vi "encoding_matlab_guoy.vi"(0 "Encoding":cluster{"d":dbl, "y0":dbl, "y1":dbl}) -> (1 "l":dbl[](array[numeric]), 2 "p":dbl[](array[numeric]), 3 "coeffs":dbl[](array[numeric]), 4 "phase":dbl[](array[numeric]))   [LabVIEW 2015]
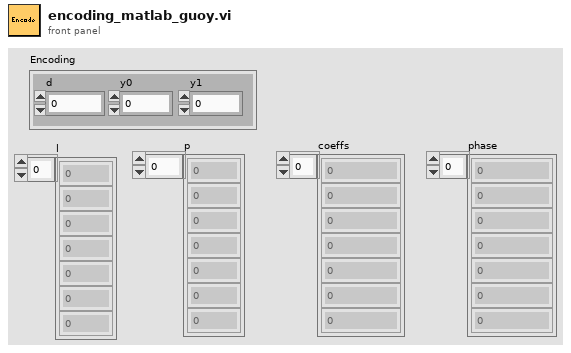
[diagram p1: front panel]
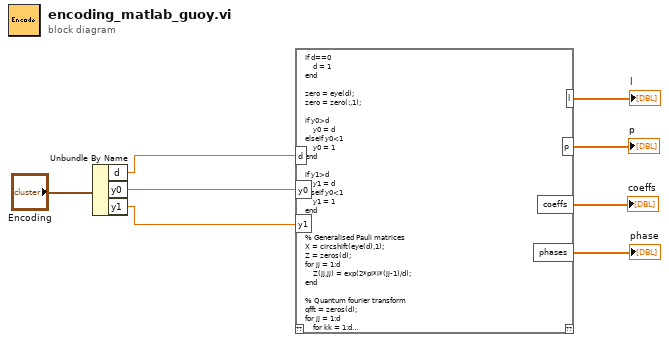
[diagram p0: block diagram]
diagram:
  n1 = Unbundle By Name("Encoding") -> ("d"=w4:dbl, "y0"=w3:dbl, "y1"=w2:dbl)
  n2 = script code="if d==0\n    d = 1\nend\n\nzero = eye(d);\nzero = zero(:,1);\n\nif y0>d \n    y0 = d\nelseif y0<1\n    y0 = 1\nend\n\nif y1>d \n    y1 = d\nelseif y0<1\n    y1 = 1\nend\n\n\n% Generalised Pauli matrices\nX = circshift(eye(d),1);\nZ = zeros(d);\nfor jj = 1:d\n    Z(jj,jj) = exp(2*pi*i*(jj-1)/d);\nend\n\n% Quantum fourier transform\nqfft = zeros(d);\nfor jj = 1:d\n    for kk = 1:d\n        qfft(jj,kk) = (1/sqrt(d))*exp(2*pi*i*(jj-1)*(kk-1)/d);\n    end\nend\n\nencode = (1/sqrt(2+(2/sqrt(d))))*(X^(y0-1))*(Z^(y1-1))*(zero+qfft*zero);\nl = [round(linspace(d-1,-d+1,d))]'\np = [(d-1-abs(l))/2]'\ncoeffs = [abs(encode)]'\nphases = [angle(encode)]'"("d"=w4, "y0"=w3, "y1"=w2) -> ("l"=→"l":dbl[], "coeffs"=→"coeffs":dbl[], "phases"=→"phase":dbl[], "p"=→"p":dbl[])  [unwired: 1 in, 1 out]
